vi "Samsung Data System.vi"(10 "Samsung String Data In":T4, 11 "Samsung Data In":u16[](array[numeric]) format="%.0x") -> (2 "Current Limit Parameters":T1 {"Min Cell Voltage Actual Value" format="%#.2f"; "Max Cell Voltage Actual Value" format="%#.2f"}, 3 "Samsung System Data Out":T2={"Voltage"=0.0, "Current"=0.0, "SOC Avg"=0.0, "Faults"=0, "Alarms"=0, "# Strings"=0, "Max Temp"=0, "Min Temp"=0, "Max Cell Voltage"=0.0, "Min Cell Voltage"=0.0, "Energy Capacity"=0.0, "Energy Remaining"=0.0, "SOC Min"=0.0, "SOC Max"=0.0, "ES Fault"=FALSE, "String Select"=enum."3 Strings", "ES Com Fault"=FALSE, "SOH Avg"=0.0})   [LabVIEW 2014]
uses:
  Controls/ES String Array.ctl
  Controls/ES String Data.ctl
  Controls/ES System Data.ctl
  Controls/StringSelector.ctl
  Controls/Current Limit Parameters.ctl
  <vilib>/Analysis/baseanly.llb/Mean (DBL).vi
  <vilib>/Analysis/NI_AALBase.lvlib
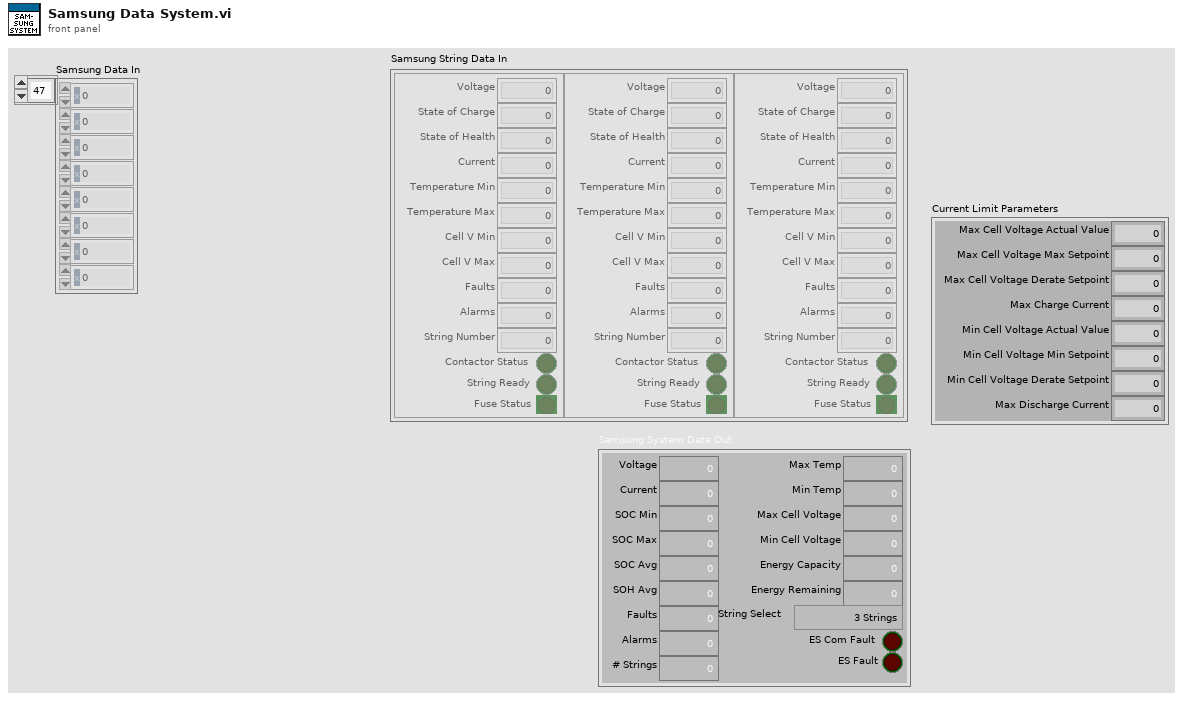
[diagram p1: front panel]
types:
  T1 = typedef "Current Limit Parameters.ctl" = cluster{"Max Cell Voltage Max Setpoint":dbl, "Max Cell Voltage Actual Value":dbl, "Max Cell Voltage Derate Setpoint":dbl, "Max Charge Current":dbl, "Min Cell Voltage Min Setpoint":dbl, "Min Cell Voltage Actual Value":dbl, "Min Cell Voltage Derate Setpoint":dbl, "Max Discharge Current":dbl}
  T2 = typedef "ES System Data.ctl" = cluster{"Voltage":sgl, "Current":sgl, "SOC Avg":sgl, "Faults":u16, "Alarms":u16, "# Strings":u16, "Max Temp":i16, "Min Temp":i16, "Max Cell Voltage":sgl, "Min Cell Voltage":sgl, "Energy Capacity":sgl, "Energy Remaining":sgl, "SOC Min":sgl, "SOC Max":sgl, "ES Fault":bool, "String Select":T3, "ES Com Fault":bool, "SOH Avg":sgl}
  T3 = typedef "StringSelector.ctl" = enum16{"1 String (1)", "1 String (2)", "1 String (3)", "2 Strings (1 2)", "2 Strings (2 3)", "2 Strings (1 3)", "3 Strings"}
  T4 = typedef "ES String Array.ctl" = T5[]
  T5 = typedef "ES String Data.ctl" = cluster{"Voltage":sgl, "State of Charge":sgl, "Current":sgl, "Temperature Min":i16, "Temperature Max":i16, "Faults":u16, "Alarms":u16, "String Number":u16, "Contactor Status":bool, "String Ready":bool, "Fuse Status":bool, "Cell V Max":dbl, "Cell V Min":dbl, "State of Health":sgl}
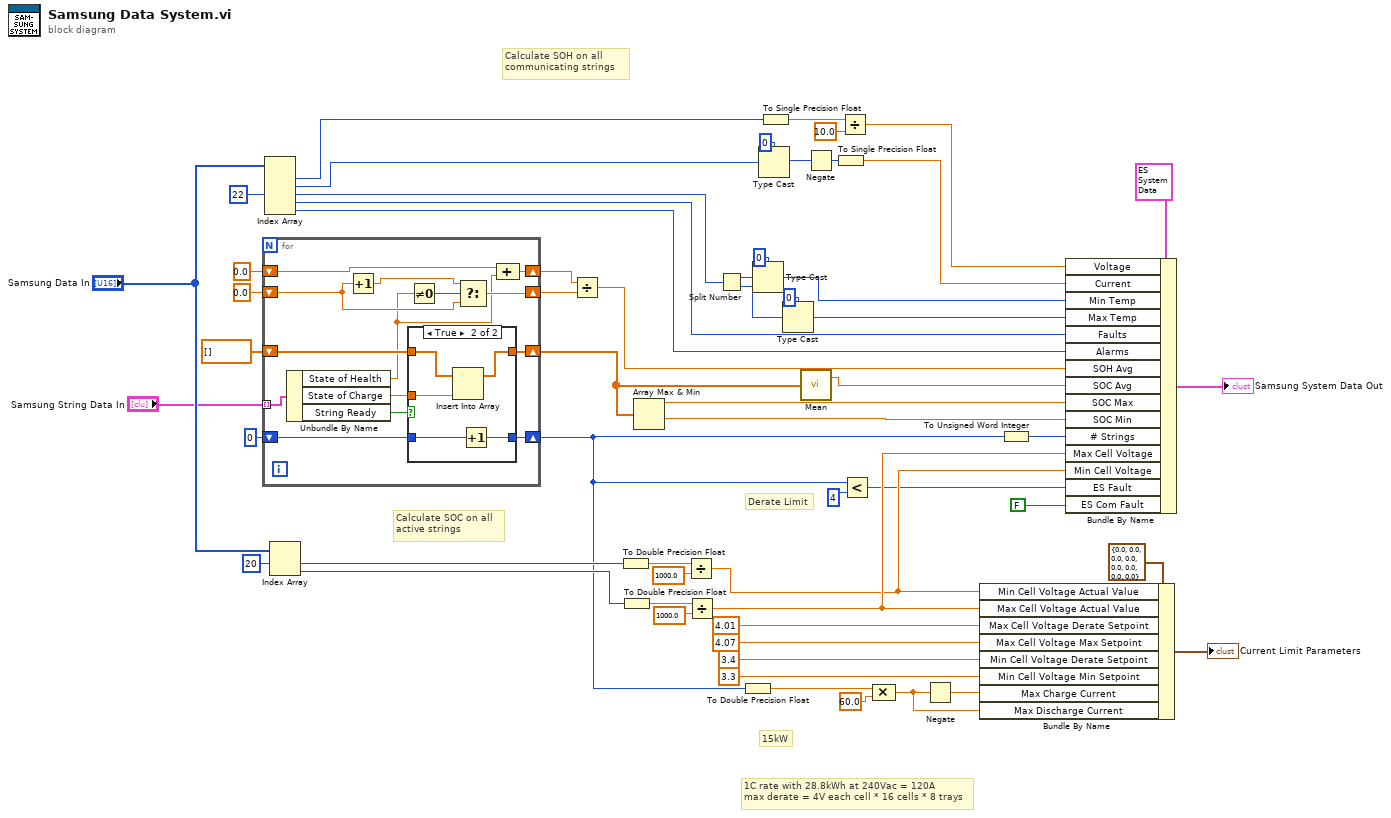
[diagram p0: block diagram]
diagram:
  # "15kW"
  # "Calculate SOC on all\nactive strings"
  # "Calculate SOH on all\ncommunicating strings"
  # "Derate Limit"
  # "1C rate with 28.8kWh at 240Vac = 120A\nmax derate = 4V each cell * 16 cells * 8 trays"
  n1 = for {
    tunnel: "Samsung String Data In" -> [w72] mode=indexing
    shift-right: [w69] -> w24
    shift-left: 0 -> [w70]
    shift-right: [w66] -> w6
    shift-left: dbl[] [] -> [w67]
    shift-right: [w64] -> w16
    shift-left: sgl 0.0 -> [w62]
    shift-right: [w60] -> w17
    shift-left: sgl 0.0 -> [w61]
    n2 = Unbundle By Name(w72) -> ("State of Health"=w59:sgl, "State of Charge"=w68:sgl, "String Ready"=w71:bool)
    n3 = Increment(x=w62) -> (x+1=w63:sgl)
    n4 = case shown="True" w71 {
      tunnel: w70 -> [w74 w79]
      tunnel: [w74 w78] -> w69
      tunnel: w68 -> [_ w76]
      tunnel: w67 -> [w73 w77]
      tunnel: [w73 w75] -> w66
      frame False {
      }
      frame True {
        n5 = Insert Into Array(array=w77, new element=w76) -> (w75:dbl[])  [unwired: 1 in]
        n6 = Increment(x=w79) -> (x+1=w78:i32)
      }
    }
    n7 = Not Equal To 0?(x=w59) -> (x != 0?=w65:bool)
    n8 = Select(t=w63, s=w65, f=w62) -> (s? t:f=w64:sgl)
    n9 = Compound Arithmetic op=ADD(w61, w59) -> (w60:sgl)
  }
  n10 = Index Array(array="Samsung Data In", index #3=22 ("index")) -> (element #1=w40:u16, element #2=w38:u16, element #3=w14:u16, element #4=w11:u16, element #5=w10:u16)  [unwired: 4 in]
  n11 = Index Array(array="Samsung Data In", index #1=20 ("index")) -> (element #1=w49:u16, element #2=w48:u16)  [unwired: 1 in]
  n12 = Divide(x=w17, y=w16) -> (x/y=w9:sgl)
  n13 = To Double Precision Float(number=w49) -> (double precision float=w54:dbl)
  n14 = To Double Precision Float(number=w48) -> (double precision float=w52:dbl)
  n15 = Array Max & Min(array=w6) -> (max value=w8:dbl, min value=w7:dbl)  [unwired: 2 out]
  n16 = Divide(x=w54, y=1000.0) -> (x/y=w31:dbl)
  n17 = Divide(x=w52, y=1000.0) -> (x/y=w32:dbl)
  n18 = Split Number(x=w14) -> (hi(x)=w21:u8, lo(x)=w33:u8)
  n19 = To Double Precision Float(number=w24) -> (double precision float=w28:dbl)
  n20 = Type Cast(type=i8 0, x=w21) -> (*(type *) &x=w13:i8)
  n21 = Type Cast(type=i16 0, x=w38) -> (*(type *) &x=w35:i16)
  n22 = To Single Precision Float(number=w40) -> (single precision float=w56:sgl)
  n23 = Type Cast(type=i8 0, x=w33) -> (*(type *) &x=w12:i8)
  n24 = call-poly <vilib>:"Mean.vi"("X"=w6) -> ("mean"=w5:dbl)  [unwired: 1 out]
  n25 = Negate(x=w35) -> (-x=w39:i16)
  n26 = To Single Precision Float(number=w39) -> (single precision float=w37:sgl)
  n27 = Divide(x=w56, y=sgl 10.0) -> (x/y=w41:sgl)
  n28 = Less?(x=w24, y=4) -> (x < y?=w2:bool)
  n29 = Compound Arithmetic op=MULTIPLY(w28, 60.0 ("value")) -> (w25:dbl)
  n30 = Negate(x=w25) -> (-x=w26:dbl)
  n31 = Bundle By Name(cluster=T1 {"Max Cell Voltage Max Setpoint"=0.0, "Max Cell Voltage Actual Value"=0.0, "Max Cell Voltage Derate Setpoint"=0.0, "Max Charge Current"=0.0, "Min Cell Voltage Min Setpoint"=0.0, "Min Cell Voltage Actual Value"=0.0, "Min Cell Voltage Derate Setpoint"=0.0, "Max Discharge Current"=0.0} ("Current Limit Parameters"), "Min Cell Voltage Actual Value"=w31, "Max Cell Voltage Actual Value"=w32, "Max Cell Voltage Derate Setpoint"=4.01 ("Max Cell Voltage Setpoint"), "Max Cell Voltage Max Setpoint"=4.07 ("Max Cell Voltage Setpoint"), "Min Cell Voltage Derate Setpoint"=3.4 ("Max Cell Voltage Setpoint"), "Min Cell Voltage Min Setpoint"=3.3 ("Max Cell Voltage Setpoint"), "Max Charge Current"=w26, "Max Discharge Current"=w25) -> (→"Current Limit Parameters":T1)
  n32 = To Unsigned Word Integer(number=w24) -> (unsigned 16bit integer=w3:u16)
  n33 = Bundle By Name(cluster=T2 {"Voltage"=0.0, "Current"=0.0, "SOC Avg"=0.0, "Faults"=0, "Alarms"=0, "# Strings"=0, "Max Temp"=0, "Min Temp"=0, "Max Cell Voltage"=0.0, "Min Cell Voltage"=0.0, "Energy Capacity"=0.0, "Energy Remaining"=0.0, "SOC Min"=0.0, "SOC Max"=0.0, "ES Fault"=FALSE, "String Select"=enum."1 String (1)", "ES Com Fault"=FALSE, "SOH Avg"=0.0} ("Energy Storage System Data"), "Voltage"=w41, "Current"=w37, "Min Temp"=w13, "Max Temp"=w12, "Faults"=w11, "Alarms"=w10, "SOH Avg"=w9, "SOC Avg"=w5, "SOC Max"=w8, "SOC Min"=w7, "# Strings"=w3, "Max Cell Voltage"=w32, "Min Cell Voltage"=w31, "ES Fault"=w2, "ES Com Fault"=FALSE) -> (→"Samsung System Data Out":T2)
